vi "channel wire.vi"() -> ()   [LabVIEW 2016]
uses:
  <extravilib>/ChannelInstances/Stream-dbl/Read With Abort.vi
  <extravilib>/ChannelInstances/Stream-dbl/Write With Abort.vi
  <extravilib>/ChannelInstances/Stream-dbl/Endpoint.vi
  <extravilib>/ChannelInstances/Stream-dbl/Instantiate.vi
  <extravilib>/ChannelInstances/Stream-dbl/)Channel.vi
  <resource>/ChannelSupport/_ChannelSupport/WaitIfNeeded.vi
  <extravilib>/ChannelInstances/Stream-dbl.lvlib
panel:
  in  "B1 2":bool
  in  "espera 2":u32
  out "indice 2":i32
  out "Waveform Chart 2":dbl(graph)
  out "Waveform Chart":dbl(graph)
  out "indice 1":i32
  in  "espera 1":u32
  in  "B1":bool
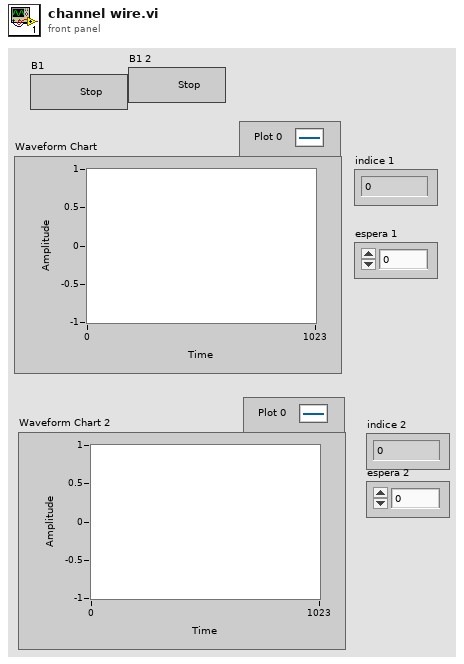
[diagram p1: front panel]
types:
  T1 = typedef "Stream-dbl.lvlib/)Channel.ctl" = refnum<queue>
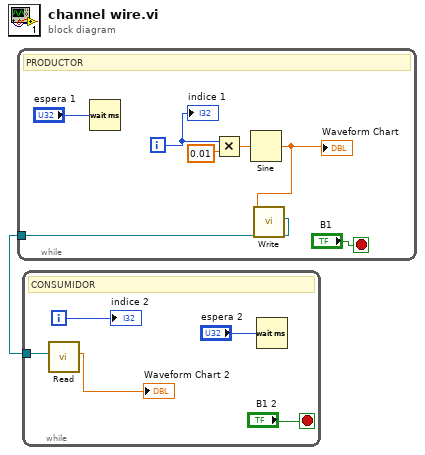
[diagram p0: block diagram]
diagram:
  n1 = while {
    tunnel: [w2] -> w1
    i -> [w6]
    stop <- "B1" stop-if-true
    # "PRODUCTOR"
    n2 = Wait (ms)(milliseconds to wait="espera 1") -> ()  [unwired: 1 out]
    n3 = Multiply(x=w6, y=0.01) -> (x*y=w5:dbl)
    n4 = Sine(x=w5) -> (sin(x)=w3:dbl)
    "Waveform Chart" <- w3
    n5 = call <extravilib>:"Write.vi"("element"=w3) -> ("channel"=w2:T1)  [unwired: 8 in, 2 out]
    "indice 1" <- w6
  }
  n6 = while {
    tunnel: w1 -> [w10]
    i -> [w12]
    stop <- "B1 2" stop-if-true
    # "CONSUMIDOR"
    n7 = call <extravilib>:"Read.vi"("channel"=w10) -> ("element"=→"Waveform Chart 2":dbl)  [unwired: 6 in, 4 out]
    n8 = Wait (ms)(milliseconds to wait="espera 2") -> ()  [unwired: 1 out]
    "indice 2" <- w12
  }
